vi "run servo.vi"(8 "错误输入（无错误）":errorcluster, 10 "hand":T1={"手腕"=52.38806, "小手指"=0.0, "无名指"=0.0, "中指"=0.0, "食指"=0.0, "上下移动"=-1.8918918918918917, "背景色"=15204350, "拇指"=0.0, "转台"=52.38806, "手臂"=52.38806} {"手臂" scale=0.0..90.0; "转台" scale=0.0..360.0; "拇指" scale=0.0..90.0; "上下移动" scale=0.0..100.0; "食指" scale=0.0..90.0; "中指" scale=0.0..90.0; "无名指" scale=0.0..90.0; "小手指" scale=0.0..90.0; "手腕" scale=0.0..360.0}, 11 "Arduino Resource输入":T2) -> (0 "错误输出":errorcluster, 3 "Arduino Resource输出":T2)   [LabVIEW 2016]
uses:
  <vilib>/LabVIEW Interface for Arduino/Type Defs/Arduino Resource.ctl
  <vilib>/LabVIEW Interface for Arduino/Type Defs/Board Type.ctl
  Controls/robotdata.ctl
  Controls/Global.vi
  <vilib>/LabVIEW Interface for Arduino/LabVIEW Interface for Arduino.lvlib
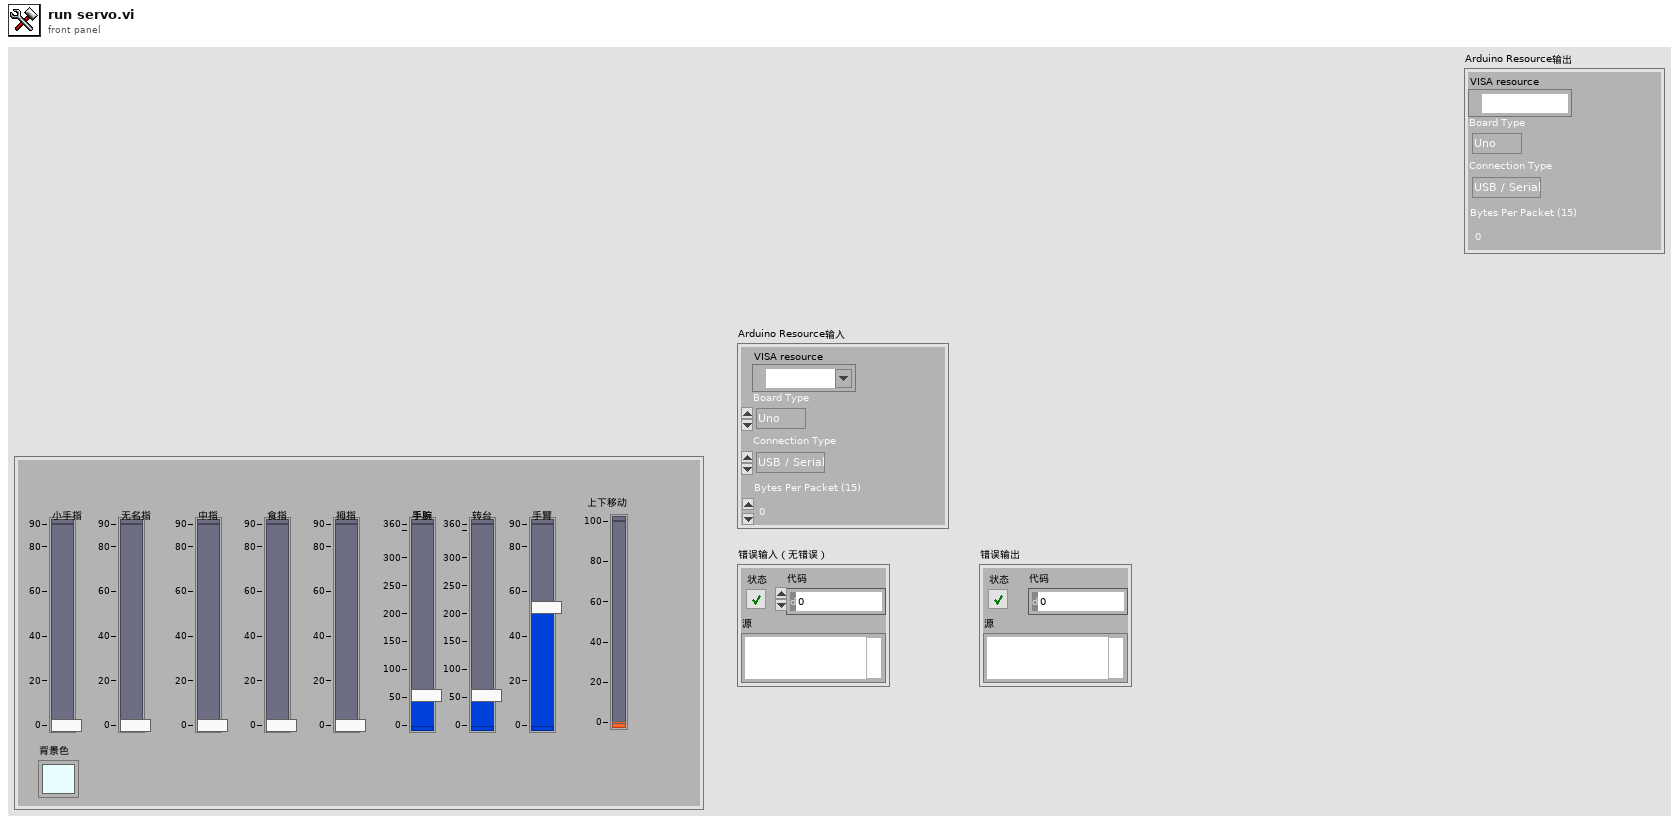
[diagram p1: front panel]
types:
  T1 = typedef "robotdata.ctl" = cluster{"手腕":sgl, "小手指":sgl, "无名指":sgl, "中指":sgl, "食指":sgl, "上下移动":dbl, "背景色":u32, "拇指":sgl, "转台":sgl, "手臂":sgl}
  T2 = typedef "LabVIEW Interface for Arduino.lvlib/Arduino Resource.ctl" = cluster{"VISA resource":refnum<visa-resource-name>, "Board Type":T3, "Connection Type":enum8{"USB / Serial"}, "Bytes Per Packet (15)":u8}
  T3 = typedef "LabVIEW Interface for Arduino.lvlib/Board Type.ctl" = enum16{"Uno", "Dimuelanove w/Atmega 328", "Mega 2560"}
  T4 = typedef "handspara.ctl" = cluster{"thumb_servo_max":u32, "thumb_servo_min":u32, "index_servo_max ":u32, "index_servo_min":u32, "middle_servo_max ":u32, "middle_servo_min":u32, "ring_servo_max":u32, "ring_servo_min":u32, "pinky_servo_max ":u32, "pinky_servo_min ":u32, "wrist_servo_max":u32, "wrist_servo_min":u32, "arm_servo_max ":u32, "arm_servo_min":u32, "rotation_servo_max ":u32, "rotation_servo_min ":u32}
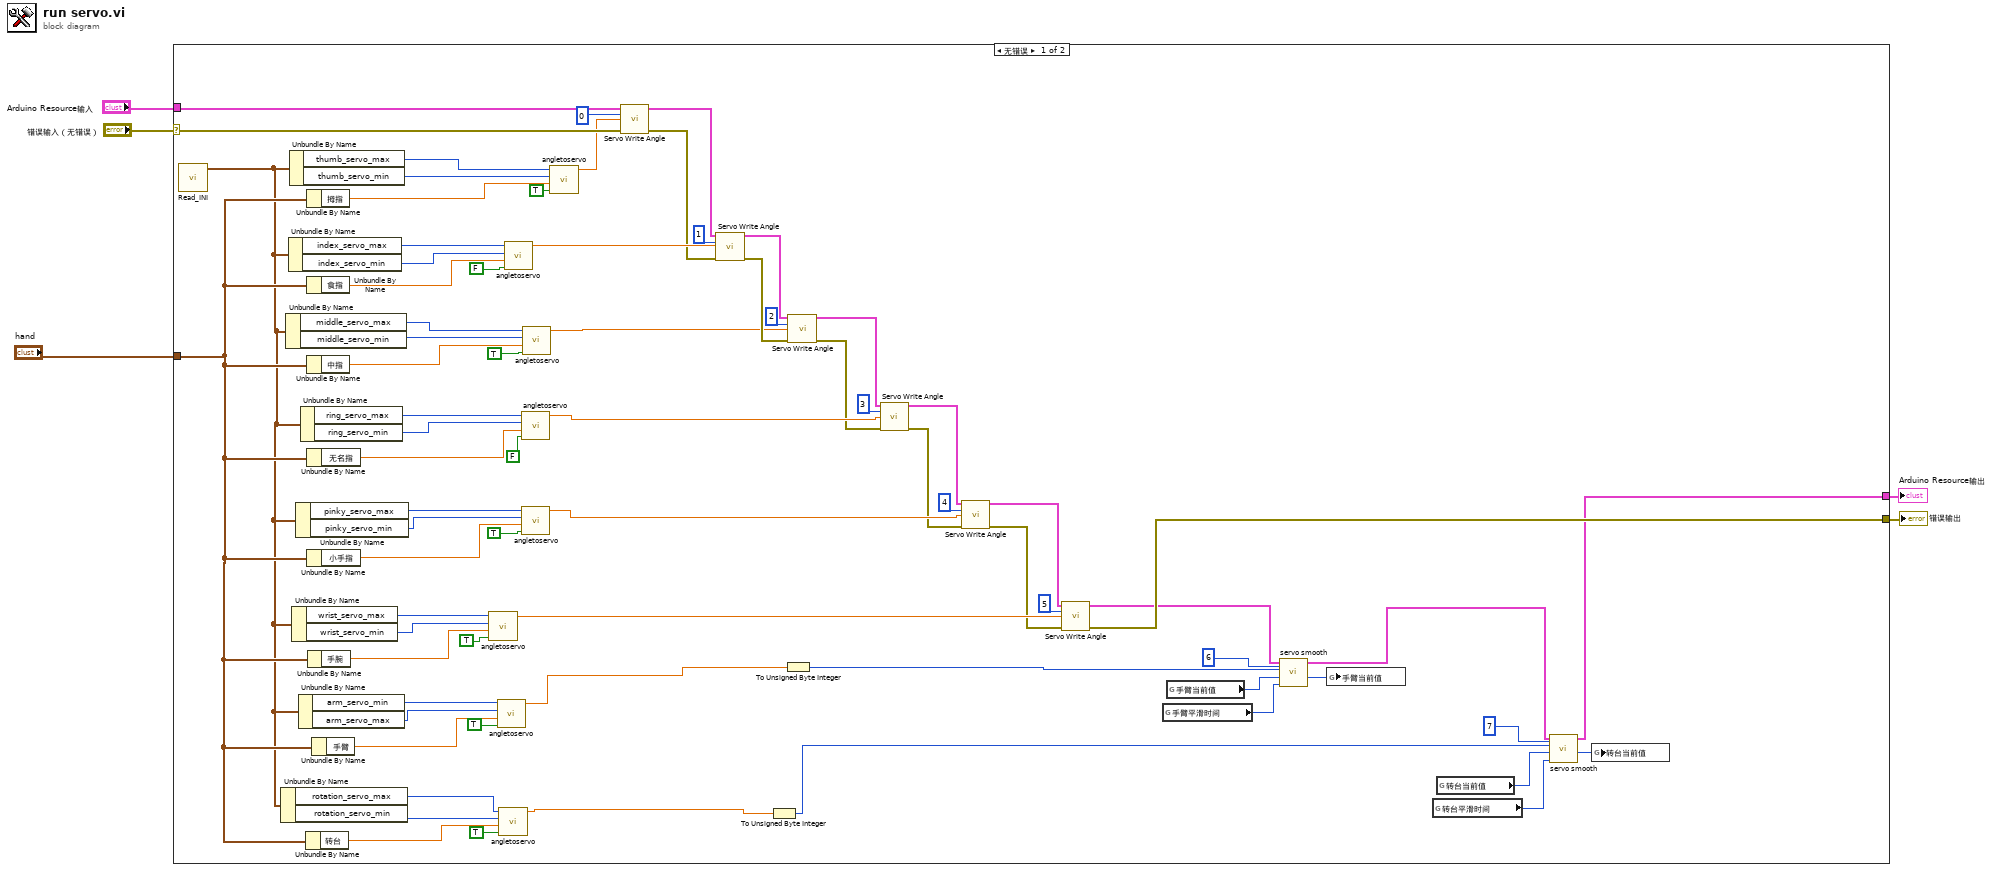
[diagram p0: block diagram]
diagram:
  n1 = case shown="无错误" "错误输入（无错误）" {
    selector: "错误输入（无错误）" -> [w71 w80]
    tunnel: "hand" -> [w20 _]
    tunnel: [w27 w80] -> w5
    tunnel: [w7 w81] -> w4
    tunnel: "Arduino Resource输入" -> [w78 w81]
    frame No Error {
      n2 = call "Read_INI.vi"() -> ("HandsPara"=w6:T4)  [unwired: 4 in, 1 out]
      n3 = Unbundle By Name(w6) -> ("rotation_servo_max"=w18:u32, "rotation_servo_min"=w17:u32)
      n4 = Unbundle By Name(w6) -> ("middle_servo_max"=w62:u32, "middle_servo_min"=w61:u32)
      n5 = Unbundle By Name(w6) -> ("index_servo_max"=w64:u32, "index_servo_min"=w63:u32)
      n6 = Unbundle By Name(w6) -> ("thumb_servo_max"=w68:u32, "thumb_servo_min"=w67:u32)
      n7 = Unbundle By Name(w6) -> ("wrist_servo_max"=w70:u32, "wrist_servo_min"=w69:u32)
      n8 = Unbundle By Name(w6) -> ("pinky_servo_max"=w66:u32, "pinky_servo_min"=w65:u32)
      n9 = Unbundle By Name(w6) -> ("arm_servo_min"=w29:u32, "arm_servo_max"=w30:u32)
      n10 = Unbundle By Name(w6) -> ("ring_servo_max"=w60:u32, "ring_servo_min"=w51:u32)
      n11 = Unbundle By Name(w20) -> ("转台"=w16:sgl)
      n12 = Unbundle By Name(w20) -> ("拇指"=w58:sgl)
      n13 = Unbundle By Name(w20) -> ("食指"=w53:sgl)
      n14 = Unbundle By Name(w20) -> ("中指"=w52:sgl)
      n15 = Unbundle By Name(w20) -> ("无名指"=w50:sgl)
      n16 = Unbundle By Name(w20) -> ("小手指"=w49:sgl)
      n17 = Unbundle By Name(w20) -> ("手腕"=w48:sgl)
      n18 = Unbundle By Name(w20) -> ("手臂"=w31:sgl)
      n19 = call "angletoservo.vi"("角度翻转"=TRUE, "手指"=w48, "最小值"=w69, "最大值输入"=w70) -> ("最大值输出"=w43:dbl)  [unwired: 7 in]
      n20 = call "angletoservo.vi"("角度翻转"=TRUE, "手指"=w31, "最小值"=w30, "最大值输入"=w29) -> ("最大值输出"=w26:dbl)  [unwired: 7 in]
      n21 = call "angletoservo.vi"("角度翻转"=TRUE, "手指"=w16, "最小值"=w17, "最大值输入"=w18) -> ("最大值输出"=w9:dbl)  [unwired: 7 in]
      n22 = call "angletoservo.vi"("角度翻转"=FALSE, "手指"=w53, "最小值"=w63, "最大值输入"=w64) -> ("最大值输出"=w56:dbl)  [unwired: 7 in]
      n23 = call "angletoservo.vi"("角度翻转"=FALSE, "手指"=w50, "最小值"=w51, "最大值输入"=w60) -> ("最大值输出"=w45:dbl)  [unwired: 7 in]
      n24 = call "angletoservo.vi"("角度翻转"=TRUE, "手指"=w49, "最小值"=w65, "最大值输入"=w66) -> ("最大值输出"=w44:dbl)  [unwired: 7 in]
      n25 = call "angletoservo.vi"("角度翻转"=TRUE, "手指"=w52, "最小值"=w61, "最大值输入"=w62) -> ("最大值输出"=w46:dbl)  [unwired: 7 in]
      n26 = call "angletoservo.vi"("角度翻转"=TRUE, "手指"=w58, "最小值"=w67, "最大值输入"=w68) -> ("最大值输出"=w59:dbl)  [unwired: 7 in]
      n27 = call <vilib>:"Servo Write Angle.vi"("Arduino Resource"=w78, "Servo Number"=u8 0, "Angle (Degrees)"=w59, "error in"=w71) -> ("Arduino Resource"=w55:T2, "error out"=w54:errorcluster)  [unwired: 10 in]
      n28 = call <vilib>:"Servo Write Angle.vi"("Arduino Resource"=w55, "Servo Number"=u8 1, "Angle (Degrees)"=w56, "error in"=w54) -> ("Arduino Resource"=w42:T2, "error out"=w47:errorcluster)  [unwired: 10 in]
      n29 = To Unsigned Byte Integer(number=w9) -> (unsigned 8bit integer=w8:u8)
      n30 = To Unsigned Byte Integer(number=w26) -> (unsigned 8bit integer=w22:u8)
      n31 = call <vilib>:"Servo Write Angle.vi"("Arduino Resource"=w42, "Servo Number"=u8 2, "Angle (Degrees)"=w46, "error in"=w47) -> ("Arduino Resource"=w40:T2, "error out"=w39:errorcluster)  [unwired: 10 in]
      n32 = call <vilib>:"Servo Write Angle.vi"("Arduino Resource"=w40, "Servo Number"=u8 3, "Angle (Degrees)"=w45, "error in"=w39) -> ("Arduino Resource"=w37:T2, "error out"=w36:errorcluster)  [unwired: 10 in]
      n33 = call <vilib>:"Servo Write Angle.vi"("Arduino Resource"=w37, "Servo Number"=u8 4, "Angle (Degrees)"=w44, "error in"=w36) -> ("Arduino Resource"=w33:T2, "error out"=w32:errorcluster)  [unwired: 10 in]
      n34 = call <vilib>:"Servo Write Angle.vi"("Arduino Resource"=w33, "Servo Number"=u8 5, "Angle (Degrees)"=w43, "error in"=w32) -> ("Arduino Resource"=w25:T2, "error out"=w27:errorcluster)  [unwired: 10 in]
      n35 = global read "Global.vi" "手臂平滑时间"() -> (w21:u32)
      n36 = global read "Global.vi" "手臂当前值"() -> (w23:u8)
      n37 = call "servo smooth.vi"("Servo Number"=u8 6, "等待时间（毫秒）"=w21, "手臂当前值输入"=w23, "servo In"=w22, "Arduino Resource"=w25) -> ("手臂当前值输出"=w12:u8, "Arduino Resource out"=w10:T2)  [unwired: 5 in]
      n38 = global write "Global.vi" "手臂当前值"(w12) -> ()
      n39 = global read "Global.vi" "转台平滑时间"() -> (w15:u32)
      n40 = global read "Global.vi" "转台当前值"() -> (w14:u8)
      n41 = call "servo smooth.vi"("Servo Number"=u8 7, "等待时间（毫秒）"=w15, "手臂当前值输入"=w14, "servo In"=w8, "Arduino Resource"=w10) -> ("手臂当前值输出"=w11:u8, "Arduino Resource out"=w7:T2)  [unwired: 5 in]
      n42 = global write "Global.vi" "转台当前值"(w11) -> ()
    }
    frame Error {
    }
  }
  "错误输出" <- w5
  "Arduino Resource输出" <- w4
